vi "delete channel from configuration.vi"(8 "error in":errorcluster, 10 "channel":refnum<class "TBM channel.lvclass">, 11 "Scan Engine configuration in":refnum<class "Scan Engine configuration.lvclass">) -> (0 "error out":errorcluster, 3 "Scan Engine configuration out":refnum<class "Scan Engine configuration.lvclass">)   [LabVIEW 2013, in "Scan Engine configuration.lvclass"]
uses:
  Scan Engine configuration.lvclass
  <vilib>/NI/Tag Bus Module Framework/channel/TBM channel.lvclass
  <vilib>/NI/Tag Bus/tag/tag descriptor.lvclass/tag descriptor.ctl
  Scan Engine configuration.lvclass/Scan Engine configuration.ctl
  <vilib>/NI/Tag Bus/tag/read tag name.vi
  <vilib>/NI/Tag Bus/tag/tag descriptor.lvclass
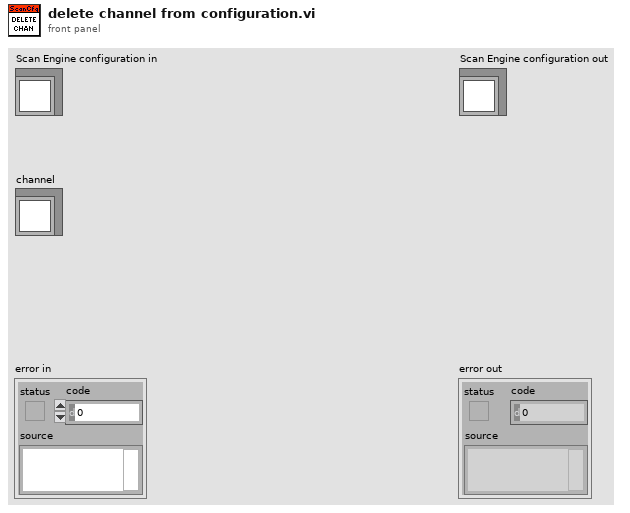
[diagram p1: front panel]
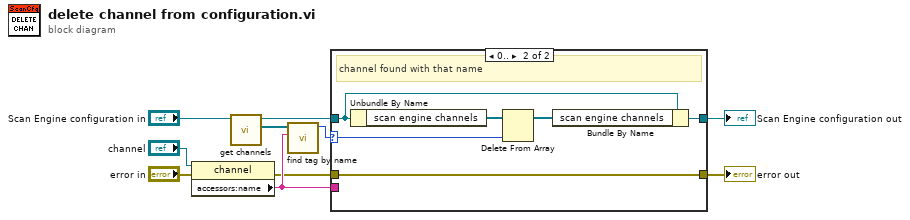
[diagram p0: block diagram]
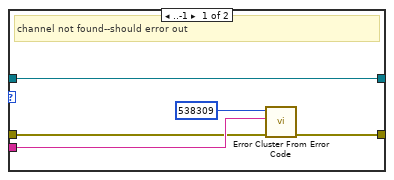
[diagram p2: hidden frame]
diagram:
  n1 = property class="channel"(reference="channel", error in="error in") -> (error out=w7:errorcluster, "accessors:name"=w9:string)  [unwired: 1 out]
  n2 = call-dynamic "get channels.vi"("module configuration in"="Scan Engine configuration in") -> ("channels"=w10:refnum<class "TBM channel.lvclass">[], "module configuration out"=w8:refnum<class "Scan Engine configuration.lvclass">)  [unwired: 9 in]
  n3 = call <vilib>:"find tag by name.vi"("name"=w9, "tags in"=w10) -> ("index"=w1:i32)  [unwired: 9 in]
  n4 = case shown="0.." w1 {
    selector: w1 -> [_ w21]
    tunnel: [w15 w16] -> w2
    tunnel: w9 -> [w13 _]
    tunnel: w7 -> [w12 w16]
    tunnel: w8 -> [w11 w19]
    tunnel: [w11 w18] -> w3
    frame ..-1 {
      # "channel not found--should error out"
      n5 = call <vilib>:"Error Cluster From Error Code.vi"("error in (no error)"=w12, "error message (\"\")"=w13, "error code (0)"=538309) -> ("error out"=w15:errorcluster)  [unwired: 6 in]
    }
    frame 0.. {
      # "channel found with that name"
      n6 = Unbundle By Name(w19) -> ("scan engine channels"=w20:refnum<class "TBM channel.lvclass">[])
      n7 = Delete From Array(array=w20, index=w21) -> (array with subset deleted=w17:refnum<class "TBM channel.lvclass">[])  [unwired: 1 in, 1 out]
      n8 = Bundle By Name(cluster=w19, "scan engine channels"=w17) -> (w18:refnum<class "Scan Engine configuration.lvclass">)
    }
  }
  "error out" <- w2
  "Scan Engine configuration out" <- w3
